vi "Close.vi"(8 "error in (no error)":errorcluster, 11 "FIFO Reader in":refnum<class "FIFO Reader.lvclass">) -> (0 "error out":errorcluster)   [LabVIEW 2024, in "RIO Streamer.lvlib" / "FIFO Reader.lvclass"]
uses:
  FIFO Reader.lvclass
  FIFO Reader.lvclass/FIFO Reader.ctl
  <vilib>/rvi/interface/nirviCloseFPGA/nirviCloseFPGA.xnode
  <vilib>/FPGAPlugInAG/Dynamic/niLvFpga_Close_Dynamic.vi
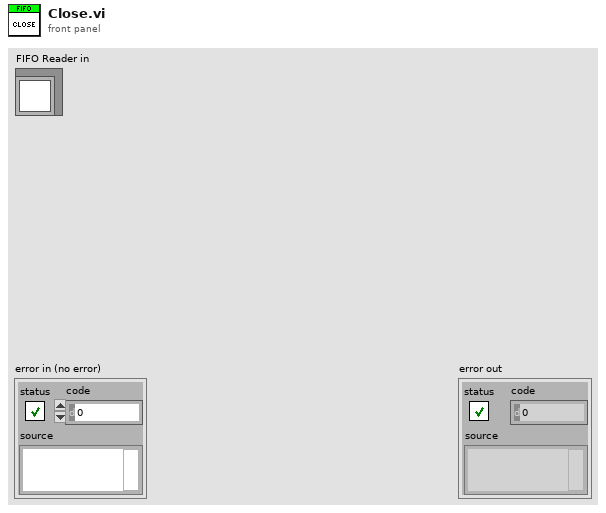
[diagram p1: front panel]
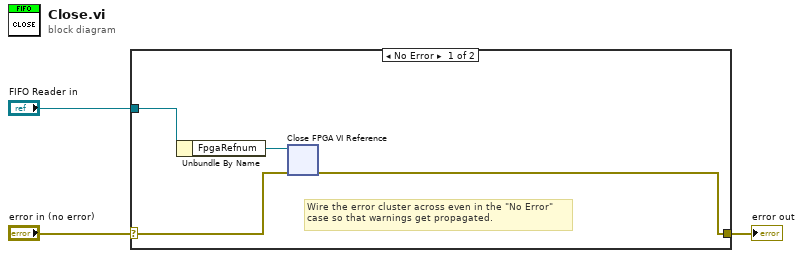
[diagram p0: block diagram]
diagram:
  n1 = case shown="No Error" "error in (no error)" {
    selector: "error in (no error)" -> [w5 w8]
    tunnel: [w4 w8] -> w2
    tunnel: "FIFO Reader in" -> [w7 _]
    frame No Error {
      # "Wire the error cluster across even in the \"No Error\"\ncase so that warnings get propagated."
      n2 = Unbundle By Name(w7) -> ("FpgaRefnum"=w6:refnum<k20>)
      n3 = xnode "Close FPGA VI Reference"("FPGA VI Reference In"=w6, "error in"=w5) -> ("error out"=w4:errorcluster)
    }
    frame Error {
    }
  }
  "error out" <- w2
